vi "4.10.1.vi"() -> ()   [LabVIEW 2018]
panel:
  out "반복 횟수":i32
  in  "정지":bool
  in  "b":bool
  in  "c":bool
  in  "a":bool
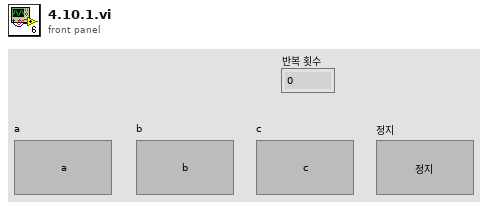
[diagram p1: front panel]
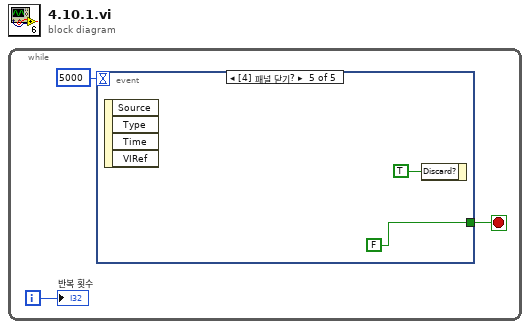
[diagram p0: block diagram]
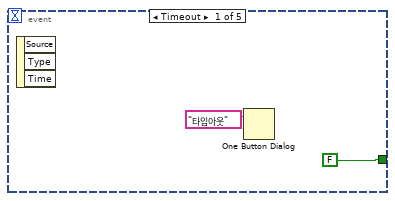
[diagram p2: hidden frame]
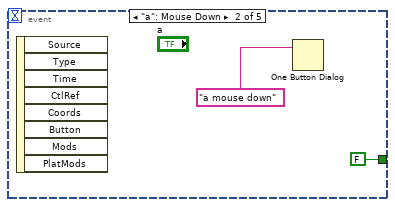
[diagram p3: hidden frame]
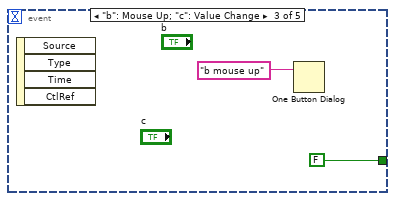
[diagram p4: hidden frame]
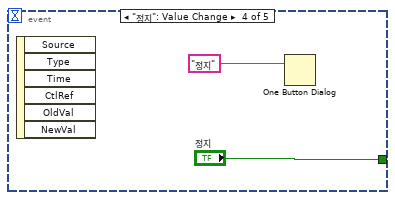
[diagram p5: hidden frame]
diagram:
  n1 = while {
    i -> [w1]
    stop <- w3 stop-if-true
    n2 = event shown="[4] 패널 닫기?" {
      selector: _ -> [_ _ _ _ _]
      dyn-events: _ -> [_ _ _ _ _]
      timeout: 5000 -> [_ _ _ _ _]
      tunnel: [FALSE FALSE ("정지") FALSE ("정지") "정지" FALSE] -> w3
      event Timeout {
        n3 = event-data() -> ()  [unwired: 1 in, 3 out]
        n4 = One Button Dialog(message="타임아웃") -> ()  [unwired: 1 in, 1 out]
      }
      event "a": Mouse Down {
        n5 = event-data() -> ()  [unwired: 1 in, 8 out]
        n6 = One Button Dialog(message="a mouse down") -> ()  [unwired: 1 in, 1 out]
      }
      event "b": Mouse Up; "c": Value Change {
        n7 = event-data() -> ()  [unwired: 1 in, 4 out]
        n8 = One Button Dialog(message="b mouse up") -> ()  [unwired: 1 in, 1 out]
      }
      event "정지": Value Change {
        n9 = event-data() -> ()  [unwired: 1 in, 6 out]
        n10 = One Button Dialog(message="정지") -> ()  [unwired: 1 in, 1 out]
      }
      event Panel Close? {
        n11 = event-data() -> ()  [unwired: 1 in, 4 out]
        n12 = event-data("Discard?"=TRUE ("버림?")) -> ()  [unwired: 1 in, 1 out]
      }
    }
    "반복 횟수" <- w1
  }
